vi "PIAxisInfoGlobal.vi"() -> ()   [LabVIEW 2011]
uses:
  PI_Axis_list.ctl
  PI_Axis.ctl
  GCS_Interface.ctl
panel:
  in  "PI GCS Function\nReferences":T1
  in  "PI Axis info":T2={"Piezo X"={"System #"=0, "Axis ID"="", "Multiplier"=1.0}, "Piezo Y"={"System #"=0, "Axis ID"="", "Multiplier"=1.0}, "Piezo Z"={"System #"=0, "Axis ID"="", "Multiplier"=1.0}, "Magnet Z"={"System #"=0, "Axis ID"="", "Multiplier"=1.0}, "Magnet Rotation"={"System #"=0, "Axis ID"="", "Multiplier"=1.0}, "Objective X"={"System #"=0, "Axis ID"="", "Multiplier"=1.0}, "Objective Y"={"System #"=0, "Axis ID"="", "Multiplier"=1.0}}
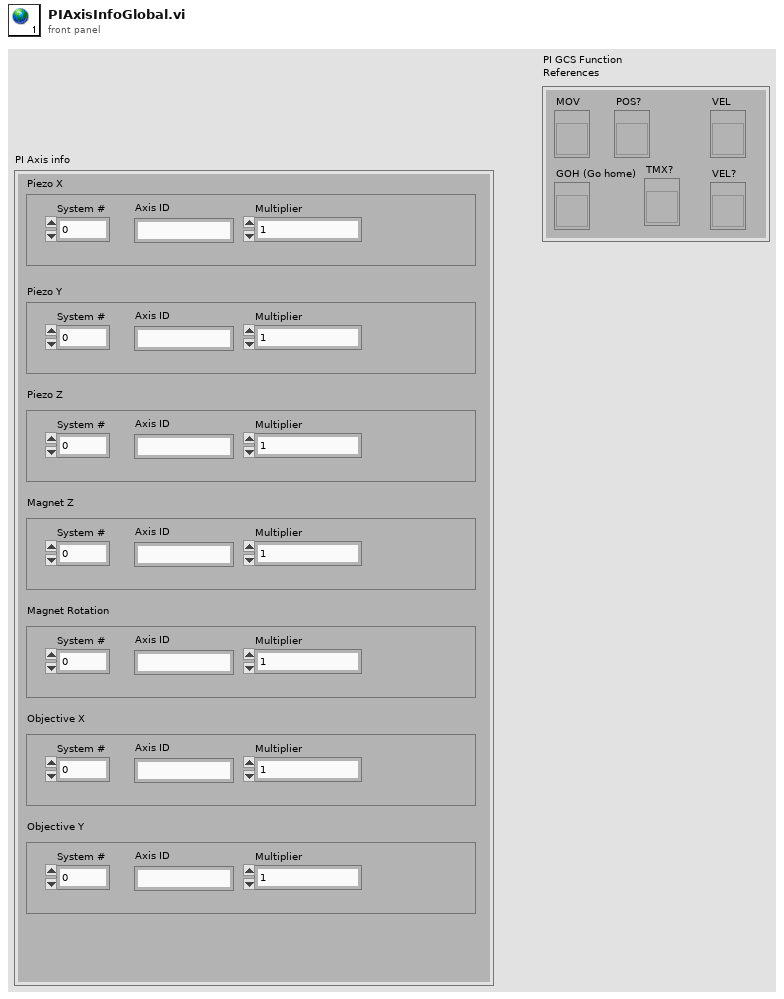
[diagram p1: front panel]
types:
  T1 = typedef "GCS_Interface.ctl" = cluster{"MOV":refnum<vi>, "VEL":refnum<vi>, "VEL?":refnum<vi>, "GOH (Go home)":refnum<vi>, "POS?":refnum<vi>, "TMX?":refnum<vi>}
  T2 = typedef "PI_Axis_list.ctl" = cluster{"Piezo X":T3, "Piezo Y":T3, "Piezo Z":T3, "Magnet Z":T3, "Magnet Rotation":T3, "Objective X":T3, "Objective Y":T3}
  T3 = typedef "PI_Axis.ctl" = cluster{"System #":i32, "Axis ID":string, "Multiplier":dbl}
diagram:
